vi "Array Max & Min Boolean.vi"(7 "JSON Array":refnum<class "JSON Array.lvclass">, 11 "error in (no error)":errorcluster) -> (4 "max value":bool, 6 "max index":i32, 8 "min value":bool, 10 "min index":i32, 15 "error out":errorcluster)   [LabVIEW 2015, in "LVJSON.lvlib" / "JSON Array.lvclass"]
uses:
  JSON Array.lvclass
  JSON Helper/To More Specific Type (Boolean).vi
  JSON Boolean/Read value (Boolean).vi
  JSON Helper/JSON Helper.lvclass
  JSON Basic Type/JSON Literal.lvclass
  JSON Boolean/JSON Boolean.lvclass
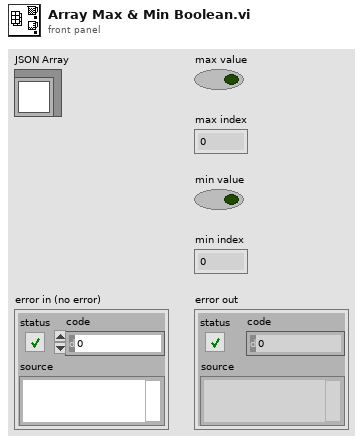
[diagram p1: front panel]
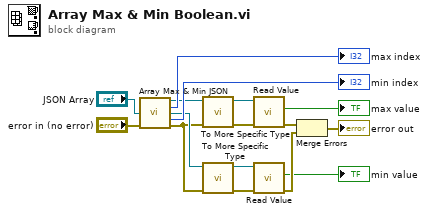
[diagram p0: block diagram]
diagram:
  n1 = call "Array Max & Min JSON.vi"("JSON Array"="JSON Array", "error in (no error)"="error in (no error)") -> ("max value"=w12:refnum<class "JSON Null.lvclass">, "max index"=→"max index":i32, "min value"=w11:refnum<class "JSON Null.lvclass">, "min index"=→"min index":i32, "error out"=w10:errorcluster)  [unwired: 9 in]
  n2 = call-poly "To More Specific Type.vi"("error in (no error)"=w10, "JSON Datatype in"=w12) -> ("error out"=w7:errorcluster, "JSON Datatype out"=w8:refnum<class "JSON Boolean.lvclass">)  [unwired: 8 in]
  n3 = call-poly "To More Specific Type.vi"("error in (no error)"=w10, "JSON Datatype in"=w11) -> ("error out"=w4:errorcluster, "JSON Datatype out"=w9:refnum<class "JSON Boolean.lvclass">)  [unwired: 8 in]
  n4 = call-poly "Read Value.vi"("error in (no error)"=w7, "JSON Boolean in"=w8) -> ("error out"=w6:errorcluster, "value"=→"max value":bool)  [unwired: 8 in]
  n5 = call-poly "Read Value.vi"("error in (no error)"=w4, "JSON Boolean in"=w9) -> ("error out"=w5:errorcluster, "value"=→"min value":bool)  [unwired: 8 in]
  n6 = Merge Errors(w6, w5) -> (→"error out":errorcluster)
